vi "get desired keys.vi"(8 "error in":errorcluster, 11 "State Machine configuration in":refnum<class "State Machine configuration.lvclass">) -> (0 "error out":errorcluster, 2 "desired keys":string[](array[string]), 3 "State Machine configuration out":refnum<class "State Machine configuration.lvclass">)   [LabVIEW 2021, in "State Machine configuration.lvclass"]
uses:
  State Machine configuration.lvclass
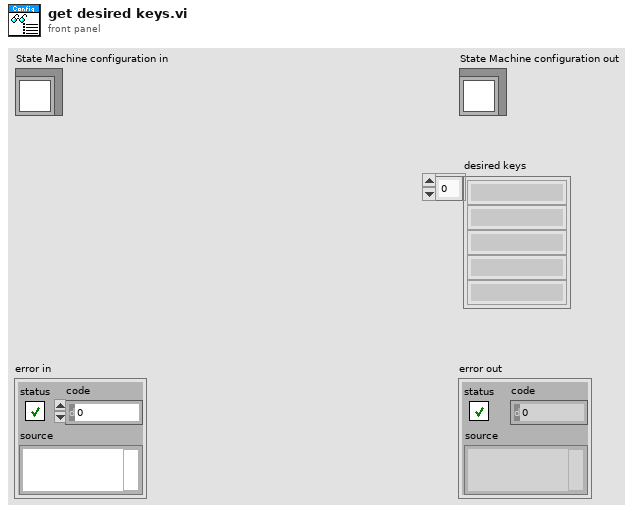
[diagram p1: front panel]
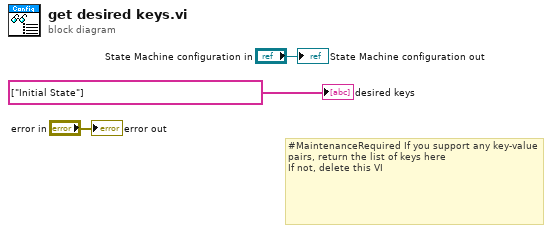
[diagram p0: block diagram]
diagram:
  # "#MaintenanceRequired If you support any key-value pairs, return the list of keys here\nIf not, delete this VI"
  "error out" <- "error in"
  "State Machine configuration out" <- "State Machine configuration in"
  "desired keys" <- string[] ["Initial State"] ("desired keys")
